vi "Close Handle.vi"(8 "error in (no error)":errorcluster, 11 "Mail in":refnum<class "Mail.lvclass">) -> (0 "error out":errorcluster, 3 "Mail out":refnum<class "Mail.lvclass">)   [LabVIEW 2023, in "HardwareAbstractionLayer_LVOOP.lvlib" / "Mail.lvclass"]
uses:
  Mail.lvclass
  Mail.lvclass/Mail.ctl
  <vilib>/smtpClient/LabVIEWSMTPClient.lvlib
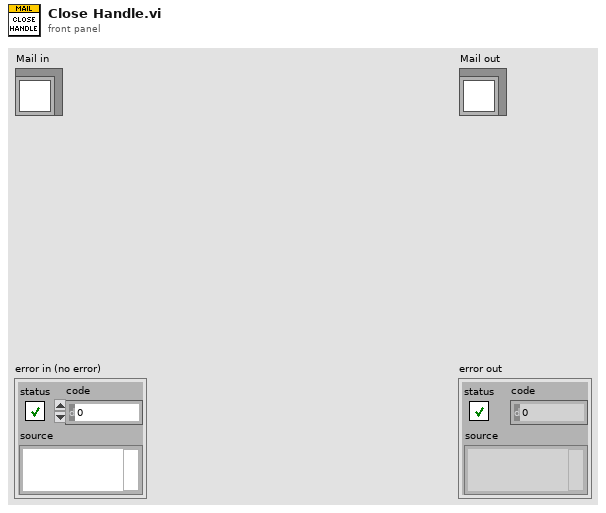
[diagram p1: front panel]
types:
  T1 = typedef "LabVIEWSMTPClient.lvlib/SmtpClientHandle.ctl" = refnum<k1>
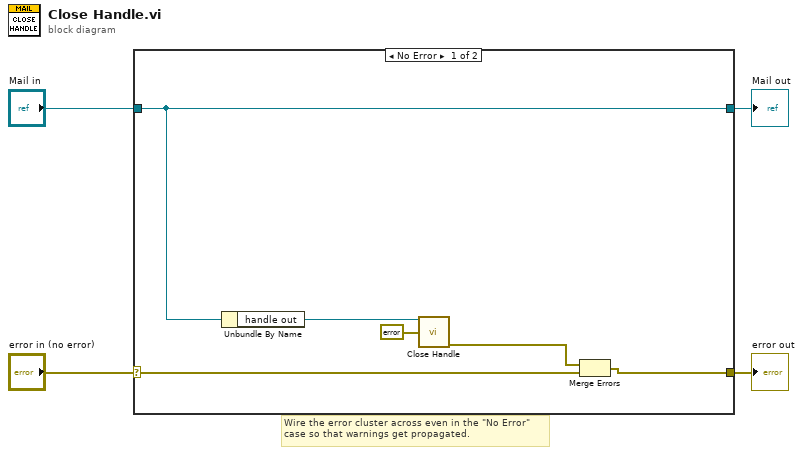
[diagram p0: block diagram]
diagram:
  # "Wire the error cluster across even in the \"No Error\"\ncase so that warnings get propagated."
  n1 = case shown="No Error" "error in (no error)" {
    selector: "error in (no error)" -> [w5 w12]
    tunnel: [w6 w12] -> w3
    tunnel: [w10 w11] -> w1
    tunnel: "Mail in" -> [w10 w11]
    frame No Error {
      n2 = Unbundle By Name(w10) -> ("handle out"=w9:T1)
      n3 = call <vilib>:"Close Handle.vi"("handle in"=w9, "error in (no error)"=errorcluster {"status"=FALSE, "code"=0, "source"=""}) -> ("error out"=w8:errorcluster)  [unwired: 12 in, 1 out]
      n4 = Merge Errors(w8, w5) -> (w6:errorcluster)
    }
    frame Error {
    }
  }
  "error out" <- w3
  "Mail out" <- w1
